vi "Build Preview.vi"(7 "Ambient":dbl, 8 "error in (no error)":errorcluster, 10 "PanelArray":refnum<class "PanelArray.lvclass">, 11 "Recipe Editor in":refnum<class "Recipe Editor.lvclass">) -> (0 "error out":errorcluster, 2 "Step Plot Data":cluster{"Time":dbl[], "Value":dbl[]}, 3 "Recipe Editor out":refnum<class "Recipe Editor.lvclass">)   [LabVIEW 2018, in "Temp Recipe.lvlib" / "Recipe Editor.lvclass"]
uses:
  Recipe Editor.lvclass
  Libraries/OOPanel/OOPanel/PanelArray/PanelArray.lvclass
  Recipe Step/Recipe Step.lvclass
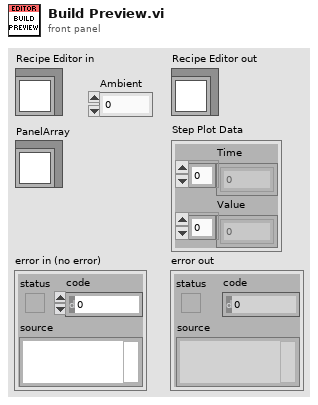
[diagram p1: front panel]
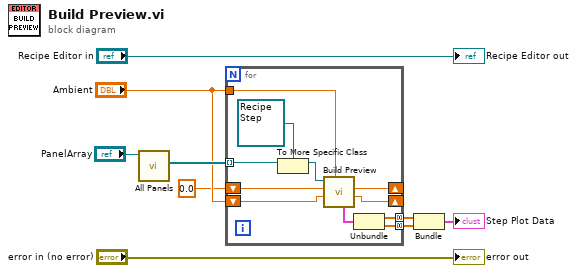
[diagram p0: block diagram]
diagram:
  n1 = call "All Panels.vi"("PanelArray in"="PanelArray") -> ("All Panels"=w6:refnum<class "Panel.lvclass">[])  [unwired: 8 in, 2 out]
  n2 = for {
    tunnel: w6 -> [w20] mode=indexing
    tunnel: "Ambient" -> [w10]
    shift-right: [w16] -> _
    shift-left: "Ambient" -> [w17]
    tunnel: [w14] -> w3 mode=concatenating
    tunnel: [w13] -> w2 mode=concatenating
    shift-right: [w11] -> _
    shift-left: 0.0 -> [w12]
    n3 = To More Specific Class(target class=refnum<class "Recipe Step.lvclass"> refnum ("Temp Recipe.lvlib:Recipe Step.lvclass"), reference=w20) -> (specific class reference=w18:refnum<class "Recipe Step.lvclass">)  [unwired: 1 in, 1 out]
    n4 = call-dynamic "Build Preview.vi"("Ambient"=w10, "Start Temp"=w17, "Start Time"=w12, "Recipe Step in"=w18) -> ("End Temp"=w16:dbl, "End Time"=w11:dbl, "Step Plot Data"=w15:cluster{"Time":dbl[], "Value":dbl[]})  [unwired: 3 in, 2 out]
    n5 = Unbundle(w15) -> ("Time"=w14:dbl[], "Value"=w13:dbl[])
  }
  n6 = Bundle("Time"=w3, "Value"=w2) -> (→"Step Plot Data":cluster{"Time":dbl[], "Value":dbl[]})  [unwired: 1 in]
  "error out" <- "error in (no error)"
  "Recipe Editor out" <- "Recipe Editor in"
